vi "Set XY Acceleration.vi"(8 "error in (no error)":errorcluster, 10 "ramp rates":dbl[](array[numeric]), 11 "Gantry 2":refnum<k24>) -> (0 "error out":errorcluster, 3 "Gantry 3":refnum<k24>)   [LabVIEW 2019]
uses:
  C:/Program Files (x86)/Aerotech/A3200/LabVIEW/2010/Bin/Aerotech.A3200.dll
  Program Files (x86)/Aerotech/A3200/LabVIEW/2010/Bin/Aerotech.A3200.dll
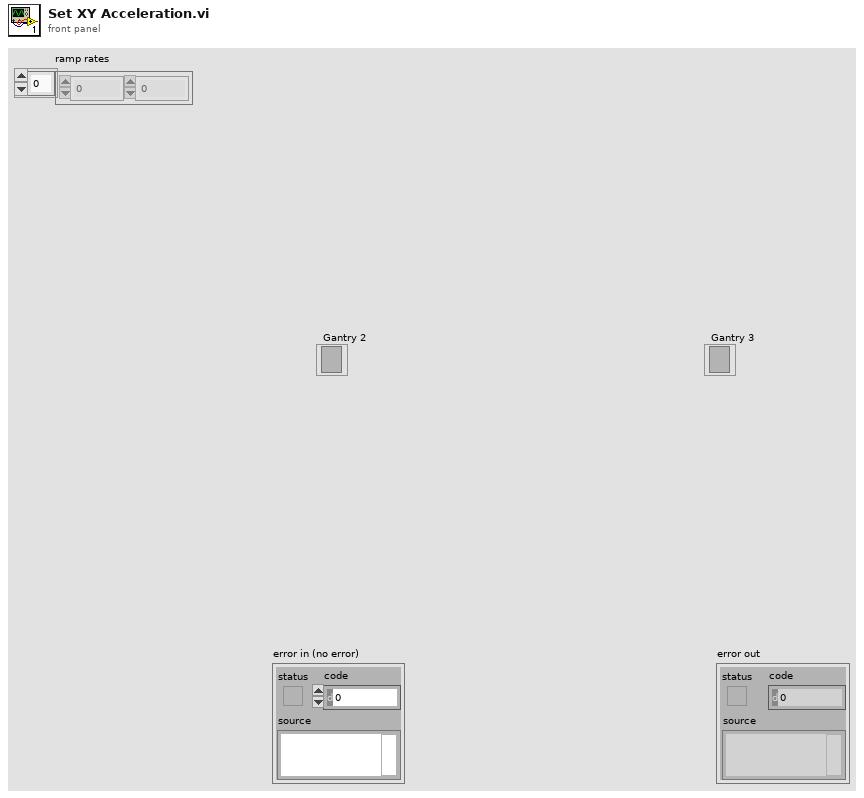
[diagram p1: front panel]
types:
  T1 = cluster{"Status":bool, "Error Code":i32, "Source":string}
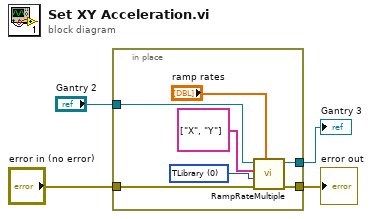
[diagram p0: block diagram]
diagram:
  n1 = in-place {
    in-place-border: "Gantry 2" -> [w10]
    in-place-border: [w9] -> w3
    in-place-border: "error in (no error)" -> [w7]
    in-place-border: [w6] -> w1
    w11 = 0 items=["TLibrary", "T01", "T02", "T03", "T04", "T05", "T06", "T07", "T08", "T09", "T10", "T11", "T12", "T13", "T14", "T15", "T16", "T17", "T18", "T19", "T20", "T21", "T22", "T23", "T24", "T25", "T26", "T27", "T28", "T29", "T30", "T31"] ("task id")
    n2 = call "RampRateMultiple.vi"("ramp rates"="ramp rates", "error in (no error)"=w7, "task id"=w11, "axis names"=string[] ["X", "Y"], "controller in"=w10) -> ("error out (no error)"=w6:T1, "controller out"=w9:refnum<k24>)  [unwired: 5 in]
  }
  "error out" <- w1
  "Gantry 3" <- w3
